vi "Increment Inspection Count.vi"(0 "Monkeys in":T1, 1 "Monkey":string) -> (3 "Monkeys out":T1)   [LabVIEW 2020, in "AoC 2022.lvlib"]
uses:
  AoC 2022.lvlib
  Monkeys.ctl
  Monkey.ctl
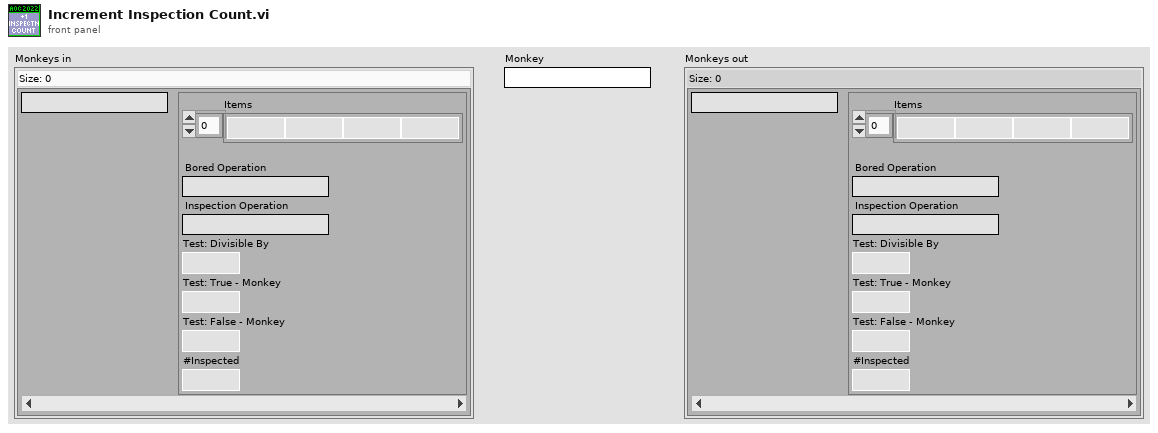
[diagram p1: front panel]
types:
  T1 = typedef "AoC 2022.lvlib/Monkeys.ctl" = map{string, T2}
  T2 = typedef "AoC 2022.lvlib/Monkey.ctl" = cluster{"Items":u64[], "Bored Operation":string, "Inspection Operation":string, "Test: Divisible By":u64, "Test: True - Monkey":i32, "Test: False - Monkey":i32, "#Inspected":i32}
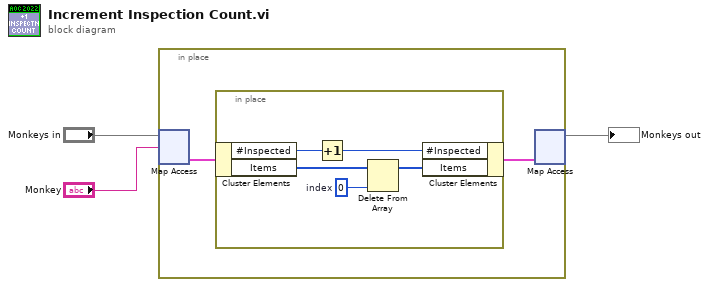
[diagram p0: block diagram]
diagram:
  n1 = in-place {
    n2 = in-place-map #1("Monkeys in", "Monkey") -> (w5:T2)  [unwired: 1 in, 1 out]
    n3 = in-place {
      w6 = 0  # index
      n4 = in-place-cluster #2(w5) -> ("#Inspected"=w10:i32, "Items"=w8:u64[])
      n5 = Increment(x=w10) -> (x+1=w9:i32)
      n6 = Delete From Array(array=w8, index=w6) -> (array with subset deleted=w7:u64[])  [unwired: 1 in, 1 out]
      n7 = in-place-cluster #2("#Inspected"=w9, "Items"=w7) -> (w4:T2)
    }
    n8 = in-place-map #1(w4) -> (→"Monkeys out":T1)  [unwired: 1 in, 2 out]
  }
